vi "GET_LayerData.vi"(8 "error in (no error)":errorcluster, 11 "Layer.lvclass in":refnum<class "Layer.lvclass">) -> (0 "error out":errorcluster, 1 "Type":T2, 2 "Data":T3={"LayerIcon"=bytes[3102], "LayerName"="", "Opacity"=100, "Visibility?"=TRUE} {"Opacity" scale=0.0..100.0}, 3 "Layer.lvclass out":refnum<class "Layer.lvclass">, 4 "Origin":T1)   [LabVIEW 2017, in "Layer.lvclass"]
doc: "Returns the User Layer Data, as well as the Type of the User Layer and the Origin."
uses:
  <vilib>/LabVIEW Icon API/lv_icon/Classes/Layer/Layer.lvclass
  <vilib>/LabVIEW Icon API/lv_icon/Controls/Layer.ctl
  <vilib>/LabVIEW Icon API/lv_icon/Controls/LayerType.ctl
  <vilib>/Utility/miscctls.llb/LVPoint32TypeDef.ctl
  <vilib>/LabVIEW Icon API/lv_icon/Classes/Layer/Layer.lvclass/Layer.ctl
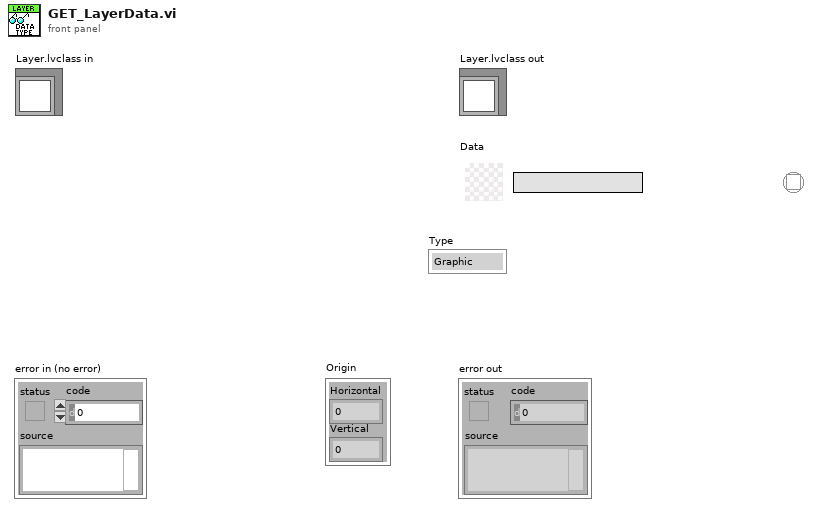
[diagram p1: front panel]
types:
  T1 = typedef "LVPoint32TypeDef.ctl" = cluster{"Horizontal":i32, "Vertical":i32}
  T2 = typedef "LayerType.ctl" = enum16{"Graphic", "Text", "Tool", "Graphic Drop"}
  T3 = typedef "Layer.ctl" = cluster{"LayerIcon":picture, "LayerName":string, "Opacity":u8, "Visibility?":bool}
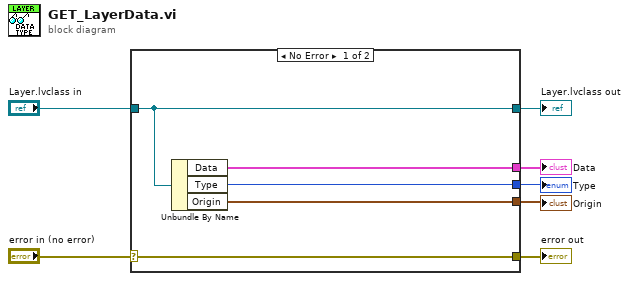
[diagram p0: block diagram]
diagram:
  n1 = case shown="No Error" "error in (no error)" {
    selector: "error in (no error)" -> [w12 w13]
    tunnel: [w12 w13] -> w6
    tunnel: [w11 w14] -> w4
    tunnel: "Layer.lvclass in" -> [w11 w14]
    tunnel: [w10 _] -> w3
    tunnel: [w9 _] -> w2
    tunnel: [w8 _] -> w1
    frame No Error {
      n2 = Unbundle By Name(w11) -> ("Data"=w10:T3, "Type"=w9:T2, "Origin"=w8:T1)
    }
    frame Error {
    }
  }
  "error out" <- w6
  "Layer.lvclass out" <- w4
  "Data" <- w3
  "Type" <- w2
  "Origin" <- w1
